vi "getScreenshot.vi"(8 "error in (no error)":errorcluster) -> (0 "error out":errorcluster, 3 "Image Data":T1)   [LabVIEW 2018, in "Image_Diff.lvlib"]
uses:
  Image_Diff.lvlib
  <vilib>/picture/picture.llb/imagedata.ctl
  System.Windows.Forms
  f295997e-83fd-4dd8-ae7b-32abe5184a50.vi
  user32.dll
panel:
  out "Screenshot":picture
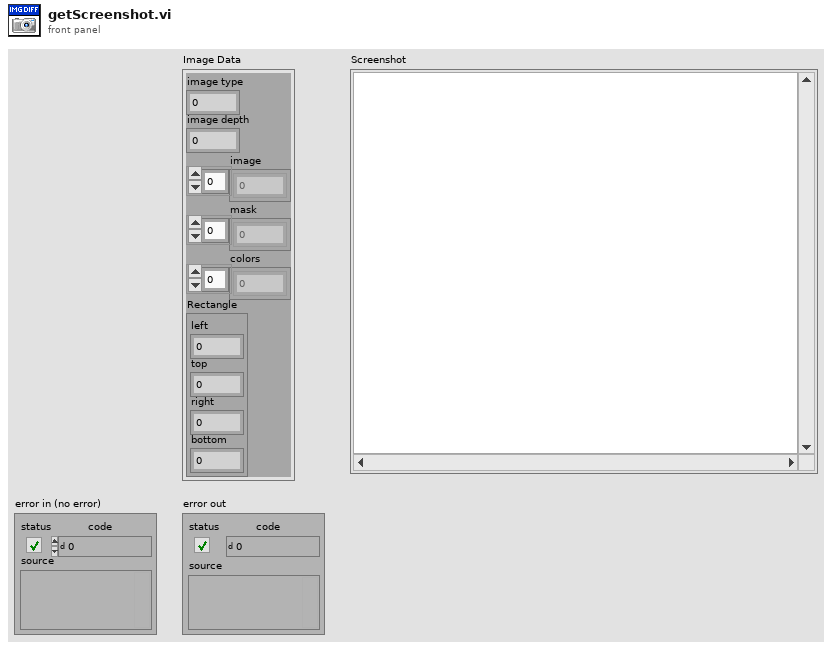
[diagram p1: front panel]
types:
  T1 = typedef "imagedata.ctl" = cluster{"image type":i32, "image depth":i32, "image":u8[], "mask":u8[], "colors":u32[], "Rectangle":cluster{"left":i16, "top":i16, "right":i16, "bottom":i16}}
  T2 = enum32{"Invalid", "Standard", "Closed", "Hidden", "Minimized", "Maximized"}
  T3 = enum16{"Left Mouse Button", "Right Mouse Button", "Ctrl-Break", "Middle Mouse Button (3-button mice only)", "X1 mouse button (Win2k Only)", "X2 Mouse Button (Win2k Only)", "Undefined (1)", "BACKSPACE", "TAB", "Reserved (1)", "Reserved (2)", "CLEAR", "ENTER", "Undefined (2)", "Undefined (3)", "SHIFT", "CTRL", "ALT", "PAUSE", "CAPS LOCK", "IME Kana mode", "Undefined (4)", "IME Junja mode", "IME final mode", "IME Hanja mode", "IME Kanji mode", "Undefined    ", "ESC", "IME convert", "IME nonconvert", "IME accept", "IME mode change request", "SPACEBAR", "PAGE UP", "PAGE DOWN", "END", "HOME", "LEFT ARROW", "UP ARROW", "RIGHT ARROW", "DOWN ARROW", "SELECT", "PRINT", "EXECUTE", "PRINT SCREEN", "INS", "DEL", "HELP"}
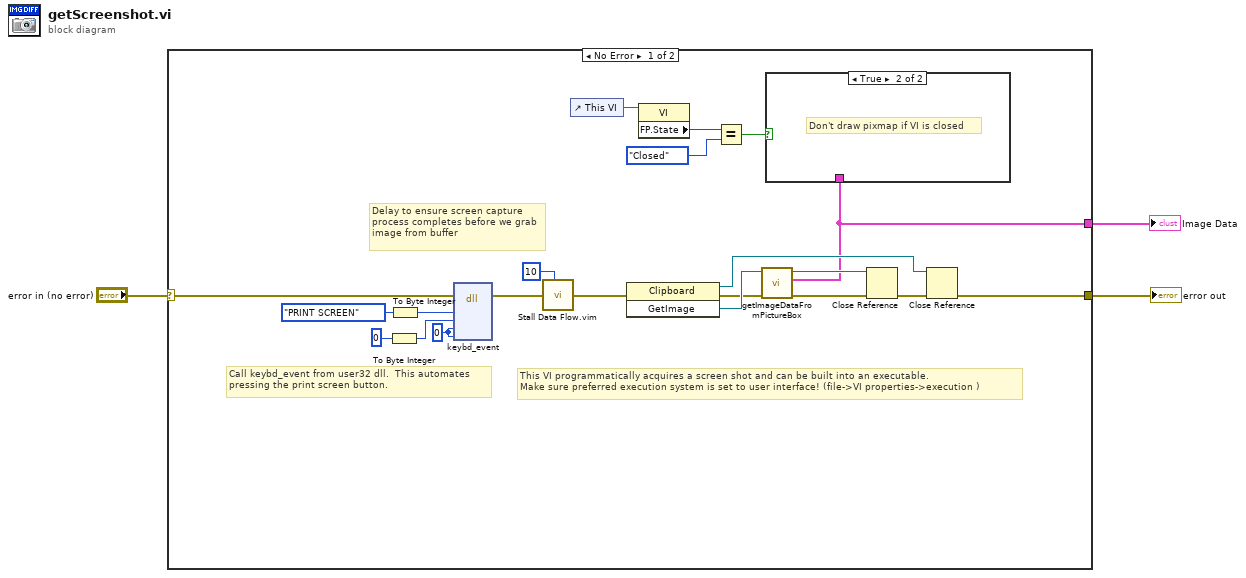
[diagram p0: block diagram]
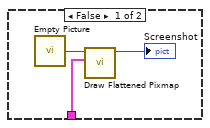
[diagram p2: hidden frame]
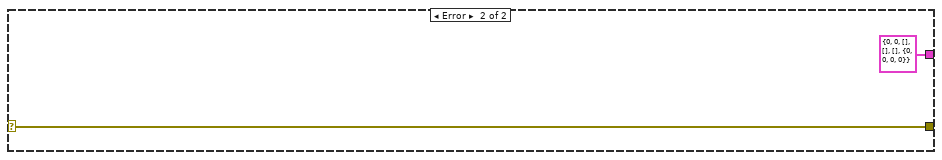
[diagram p3: hidden frame]
diagram:
  n1 = case shown="No Error" "error in (no error)" {
    selector: "error in (no error)" -> [w9 w29]
    tunnel: [w10 w29] -> w3
    tunnel: [w5 T1 {"image type"=0, "image depth"=0, "image"=[], "mask"=[], "colors"=[], "Rectangle"={"left"=0, "top"=0, "right"=0, "bottom"=0}} ("Image Data")] -> w1
    frame No Error {
      w24 = 0 ("Input Value")
      # "Delay to ensure screen capture process completes before we grab image from buffer"
      # "This VI programmatically acquires a screen shot and can be built into an executable. \nMake sure preferred execution system is set to user interface! (file->VI properties->execution )"
      # "Call keybd_event from user32 dll.  This automates\npressing the print screen button."
      n2 = To Byte Integer(number=i8 0) -> (8bit integer=w22:i8)
      n3 = To Byte Integer(number=T3."PRINT SCREEN" ("Keyboard Stroke")) -> (8bit integer=w20:i8)
      n4 = dll-call lib="user32.dll" fn="keybd_event"(error in=w9, w20, w22, w24, w24) -> (error out=w19:errorcluster)  [unwired: 7 in, 1 out]
      n5 = call "Stall Data Flow.vim"("value in"=w19, "milliseconds to wait"=u32 10) -> ("value out"=w17:errorcluster)  [unwired: 1 out]
      n6 = control-ref of="This VI"() -> (w8:refnum<vi>)
      n7 = invoke class="Clipboard" method="GetImage"(error in=w17) -> (reference out=w14:refnum<k24>, error out=w15:errorcluster, "GetImage"=w16:refnum<k24>)  [unwired: 2 in]
      n8 = property class="VI"(reference=w8) -> ("FP.State"=w7:T2)  [unwired: 1 in, 2 out]
      n9 = Equal?(x=w7, y=T2."Closed") -> (x = y?=w4:bool)
      n10 = call "getImageDataFromPictureBox.vi"("error in (no error)"=w15, "Image"=w16) -> ("error out"=w13:errorcluster, "Image Data"=w5:T1, "Image Out"=w11:refnum<k24>)  [unwired: 7 in]
      n11 = case shown="True" w4 {
        tunnel: w5 -> [w26 _]
        frame False {
          n12 = call "Empty Picture"() -> ("empty picture"=w27:picture)
          n13 = call <vilib>:"Draw Flattened Pixmap.vi"("image data"=w26, "picture"=w27) -> ("new picture"=→"Screenshot":picture)  [unwired: 7 in]
        }
        frame True {
          # "Don't draw pixmap if VI is closed"
        }
      }
      n14 = Close Reference(reference=w11, error in (no error)=w13) -> (error out=w12:errorcluster)
      n15 = Close Reference(reference=w14, error in (no error)=w12) -> (error out=w10:errorcluster)
    }
    frame Error {
    }
  }
  "error out" <- w3
  "Image Data" <- w1
